vi "Try Start Video.vi"(8 "error in (no error)":errorcluster, 11 "SB App in":refnum<class "SB App.lvclass">) -> (0 "error out":errorcluster, 3 "SB App out":refnum<class "SB App.lvclass">)   [LabVIEW 2020, in "SB App.lvlib" / "SB App.lvclass"]
uses:
  SB App.lvclass
  SB App.lvclass/SB App.ctl
  <vilib>/Utility/sysdir.llb/System Directory Type.ctl
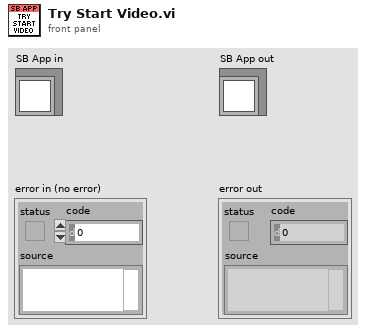
[diagram p1: front panel]
types:
  T1 = typedef "System Directory Type.ctl" = i32
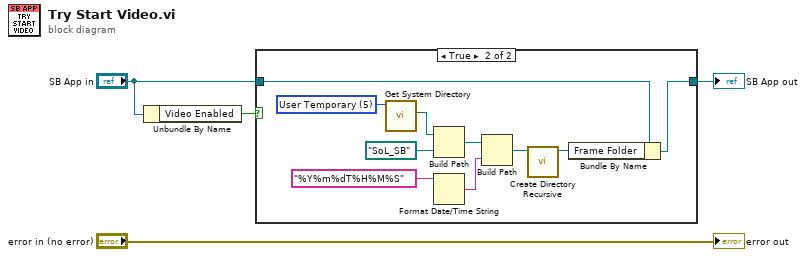
[diagram p0: block diagram]
diagram:
  n1 = Unbundle By Name("SB App in") -> ("Video Enabled"=w4:bool)
  n2 = case shown="True" w4 {
    tunnel: "SB App in" -> [w5 w8]
    tunnel: [w5 w6] -> w2
    frame False {
    }
    frame True {
      w15 = T1 5 items=["User Home"=0, "User Desktop"=1, "User Documents"=2, "User Application Data"=3, "User Preferences"=4, "User Temporary"=5, "Public Documents"=6, "Public Application Data"=7, "Public Preferences"=8, "Public Cache"=13, "System Core Libraries"=9, "System Installed Libraries"=10, "Application Files"=11, "Boot Volume Root"=12] ("system directory type")
      n3 = call <vilib>:"Get System Directory.vi"("system directory type"=w15) -> ("system directory"=w14:path)  [unwired: 10 in]
      n4 = Build Path(base path=w14, name or relative path=path "SoL_SB") -> (appended path=w11:path)
      n5 = Format Date/Time String(time format string (%c)="%Y%m%dT%H%M%S") -> (date/time string=w10:string)  [unwired: 2 in]
      n6 = Build Path(base path=w11, name or relative path=w10) -> (appended path=w9:path)
      n7 = call <vilib>:"Create Directory Recursive.vi"("directory"=w9) -> ("directory copy"=w7:path)  [unwired: 4 in, 2 out]
      n8 = Bundle By Name(cluster=w8, "Frame Folder"=w7) -> (w6:refnum<class "SB App.lvclass">)
    }
  }
  "SB App out" <- w2
  "error out" <- "error in (no error)"
